vi "Calc_Anchor_Posi.vi"(8 "Initial Anchor Position":dbl[][](array[numeric]), 11 "Center State at T":T1) -> (3 "Anchor Posi at T":dbl[][](array[numeric]))   [LabVIEW 2020]
uses:
  <vilib>/Analysis/baseanly.llb/Mean (DBL).vi
  <vilib>/Analysis/coordinate.llb/2D Cartesian Coordinate Rotation (Array).vi
  <vilib>/Analysis/NI_AALBase.lvlib
  <vilib>/Analysis/NI_AALPro.lvlib
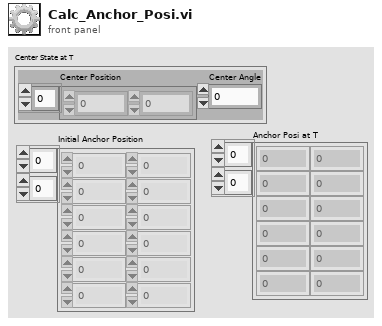
[diagram p1: front panel]
types:
  T1 = cluster{"Center Position":dbl[], "Center Angle":dbl}
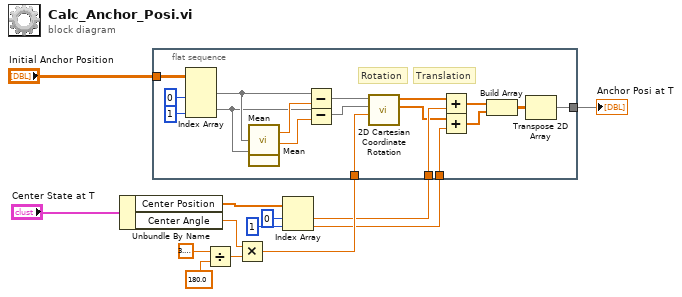
[diagram p0: block diagram]
diagram:
  n1 = Unbundle By Name("Center State at T") -> ("Center Position"=w7:dbl[], "Center Angle"=w9:dbl)
  n2 = flat-sequence {
    tunnel: w8 -> [w31]
    tunnel: [w30] -> w4
    tunnel: "Initial Anchor Position" -> [w27]
    tunnel: w2 -> [w26]
    tunnel: w1 -> [w25]
    frame #0 {
      # "Translation"
      # "Rotation"
      n3 = Index Array(array=w27, index (col) #1=0 ("disabled index (col)"), index (col) #2=1 ("index (col)")) -> (element #1=w15:dbl[], element #2=w14:dbl[])  [unwired: 2 in]
      n4 = call-poly <vilib>:"Mean.vi"("X"=w15) -> ("mean"=w19:dbl)  [unwired: 1 out]
      n5 = call-poly <vilib>:"Mean.vi"("X"=w14) -> ("mean"=w18:dbl)  [unwired: 1 out]
      n6 = Subtract(x=w15, y=w19) -> (x-y=w23:dbl[])
      n7 = Subtract(x=w14, y=w18) -> (x-y=w22:dbl[])
      n8 = call-poly <vilib>:"2D Cartesian Coordinate Rotation.vi"("theta"=w31, "Y"=w22, "X"=w23) -> ("Y Out"=w20:dbl[], "X Out"=w21:dbl[])  [unwired: 6 in, 1 out]
      n9 = Add(x=w21, y=w26) -> (x+y=w29:dbl[])
      n10 = Add(x=w20, y=w25) -> (x+y=w28:dbl[])
      n11 = Build Array(w29, w28) -> (w24:dbl[][])
      n12 = Transpose 2D Array(2D array=w24) -> (transposed array=w30:dbl[][])
    }
  }
  n13 = Divide(x=3.141592653589793, y=180.0) -> (x/y=w10:dbl)
  n14 = Multiply(x=w9, y=w10) -> (x*y=w8:dbl)
  n15 = Index Array(array=w7, index #1=0 ("index"), index #2=1 ("index")) -> (element #1=w2:dbl, element #2=w1:dbl)
  "Anchor Posi at T" <- w4
